vi "Arduino Generate Command String.vi"(10 "Filter Wheel Settings":T1={"Direction"=TRUE, "NUMBER OF  STEPS"=13000, "SPEED STEPS/SEC"=1000, "ACC/DECEL STEPS/SEC^2"=1000, "Move mode"=0, "EN/DIS?"=TRUE, "delay before \nread (ms)"=750, "Timeout before \nstop (ms)"=13000} {"Move mode" items=["Relative steps ##", "Search switch"]; "ACC/DECEL STEPS/SEC^2" max=4000; "SPEED STEPS/SEC" min=20 max=4000 step=10}, 11 "MOTOR NUMBER":u8 max=3 step=1) -> (3 "Cmd String":string)   [LabVIEW 2021, in "FW Arduino Control.lvclass"]
uses:
  FW Arduino Control.lvclass
  Filter Wheel Arduino Command cluster.ctl
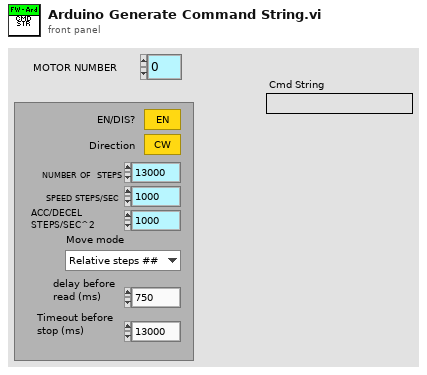
[diagram p1: front panel]
types:
  T1 = typedef "Filter Wheel Arduino Command cluster.ctl" = cluster{"Direction":bool, "NUMBER OF  STEPS":u32, "SPEED STEPS/SEC":u16, "ACC/DECEL STEPS/SEC^2":u16, "Move mode":u16, "EN/DIS?":bool, "delay before \nread (ms)":u32, "Timeout before \nstop (ms)":u32}
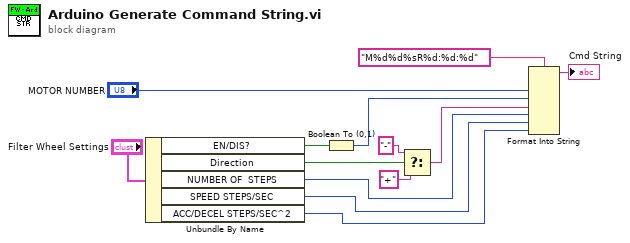
[diagram p0: block diagram]
diagram:
  n1 = Unbundle By Name("Filter Wheel Settings") -> ("EN/DIS?"=w10:bool, "Direction"=w8:bool, "NUMBER OF  STEPS"=w4:u32, "SPEED STEPS/SEC"=w3:u16, "ACC/DECEL STEPS/SEC^2"=w2:u16)
  n2 = Boolean To (0,1)(Boolean=w10) -> (0, 1=w9:i16)
  n3 = Select(t="-", s=w8, f="+") -> (s? t:f=w5:string)
  n4 = Format Into String(format string="M%d%d%sR%d:%d:%d", "MOTOR NUMBER", w9, w5, w4, w3, w2) -> (resulting string=→"Cmd String":string)  [unwired: 2 in, 1 out]
